vi "GetLastError.vi"(8 "error in (no error)":errorcluster) -> (0 "error out":errorcluster, 3 "function return":string)   [LabVIEW 2015, in "ReDeX.lvlib"]
doc: "const char* redex_lv_get_last_error(void);"
uses:
  ReDeX.lvlib
  C:/ReDeX/ReDeX.dll
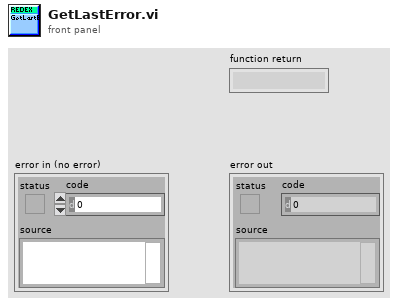
[diagram p1: front panel]
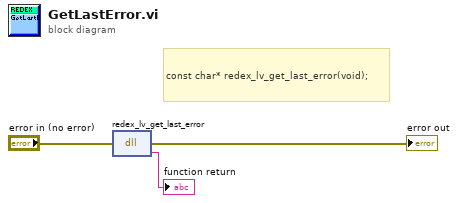
[diagram p0: block diagram]
diagram:
  # "const char* redex_lv_get_last_error(void);"
  n1 = dll-call lib="C:/ReDeX/ReDeX.dll" fn="redex_lv_get_last_error"(error in="error in (no error)") -> (error out=→"error out":errorcluster, "return type"=→"function return":string)  [unwired: 2 in, 1 out]
